vi "Producer:Consumer_UI.vi"() -> ()   [LabVIEW 2023]
panel:
  out "평가 데이터":string
  out "분석 데이터":bool
  out "측정 데이터":i32[](array[numeric])
  in  "종료":bool
  in  "평가":bool
  in  "분석":bool
  in  "측정":bool
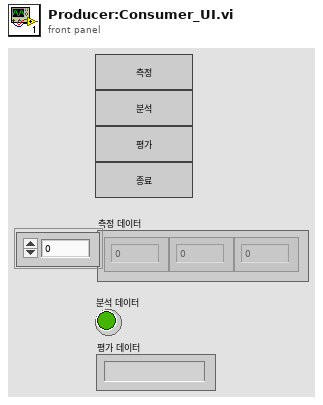
[diagram p1: front panel]
types:
  T1 = typedef "상태.ctl" = enum16{"측정", "분석", "평가", "종료"}
  T2 = enum8{"Enabled", "Disabled", "Disabled and Grayed Out"}
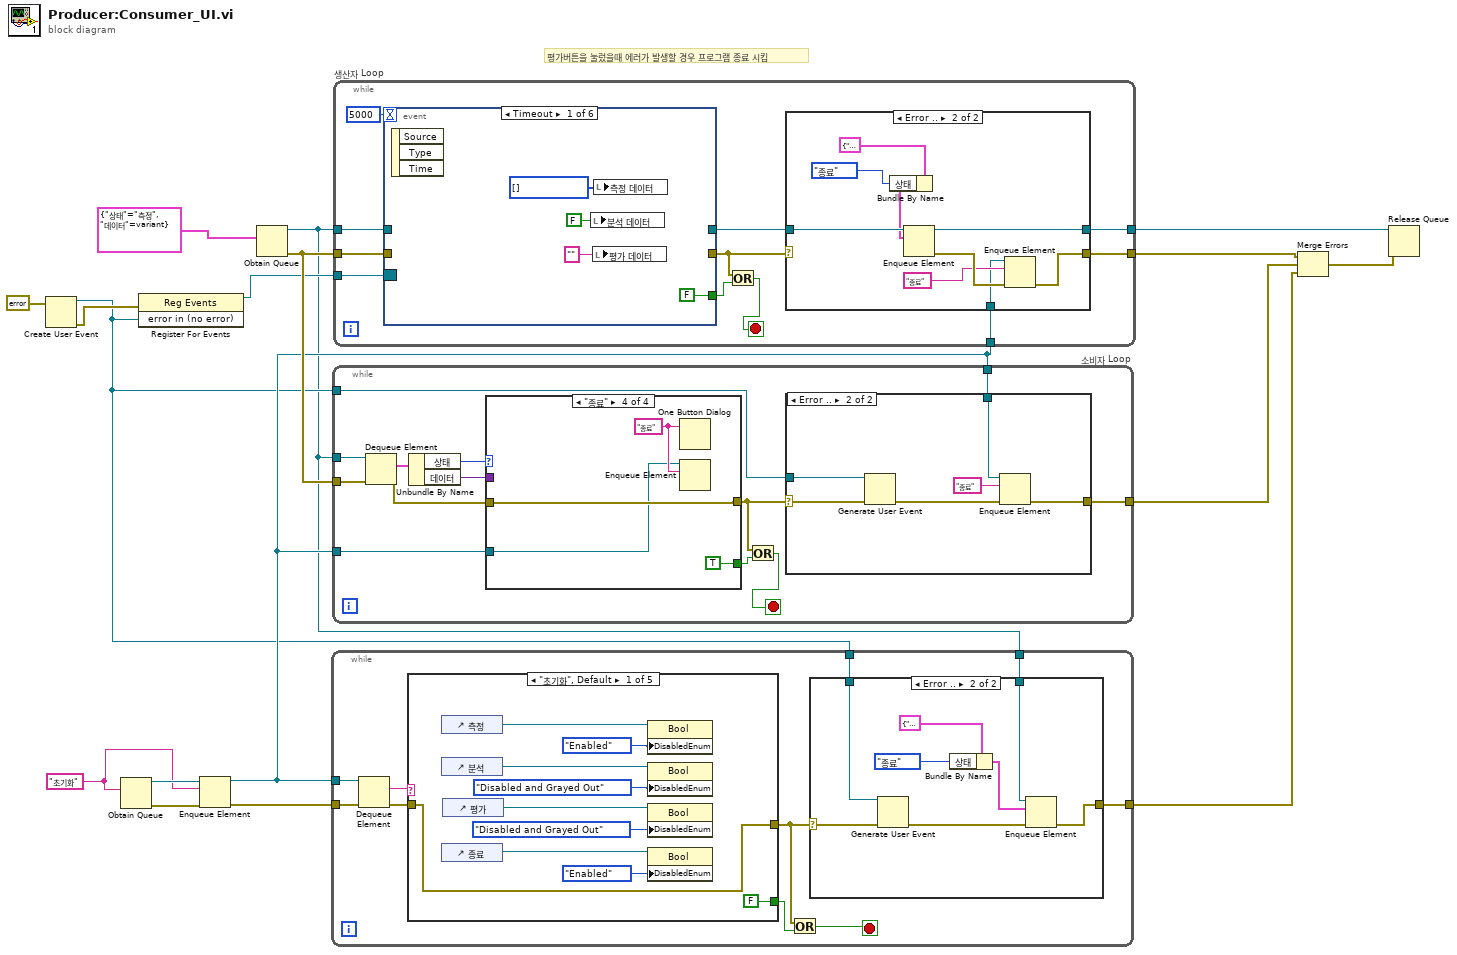
[diagram p0: block diagram]
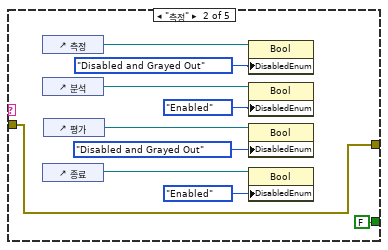
[diagram p3: hidden frame]
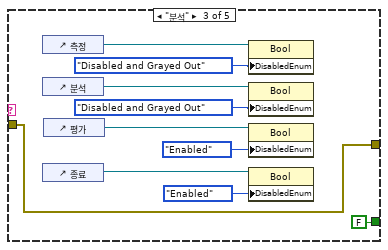
[diagram p4: hidden frame]
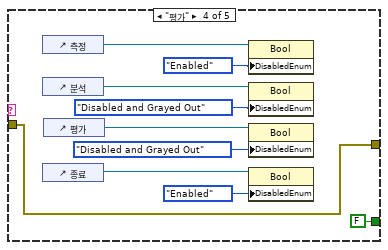
[diagram p5: hidden frame]
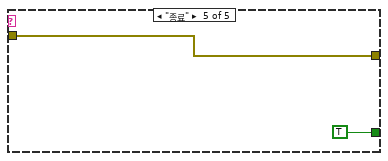
[diagram p6: hidden frame]
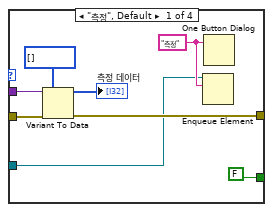
[diagram p8: hidden frame]
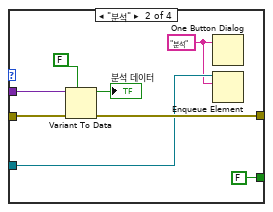
[diagram p9: hidden frame]
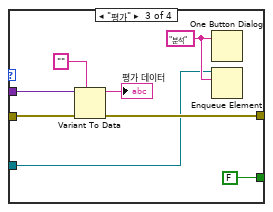
[diagram p10: hidden frame]
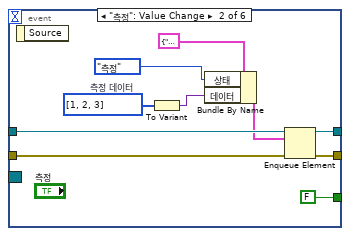
[diagram p12: hidden frame]
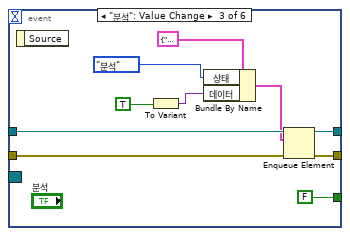
[diagram p13: hidden frame]
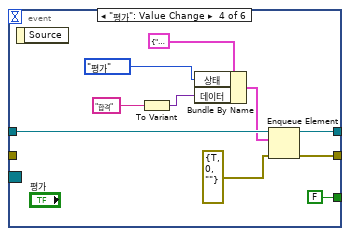
[diagram p14: hidden frame]
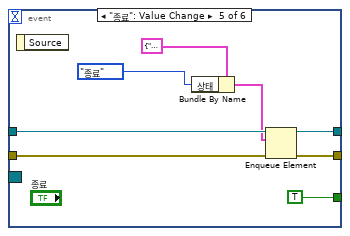
[diagram p15: hidden frame]
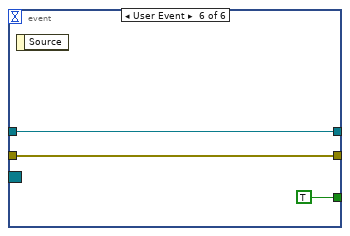
[diagram p16: hidden frame]
diagram:
  w1 = "초기화" ("name (unnamed)")
  # "평가버튼을 눌렀을때 에러가 발생할 경우 프로그램 종료 시킴"
  n1 = Create User Event(user event datatype=errorcluster {"status"=FALSE, "code"=0, "source"=""} ("error in (no error)")) -> (user event=w3:refnum<user-event>, error out=w10:errorcluster)  [unwired: 1 in]
  n2 = Obtain Queue(element data type=w1) -> (queue out=w8:refnum<queue>, error out=w7:errorcluster)  [unwired: 4 in, 1 out]
  n3 = register-events(error in=w10, w3) -> (reference out=w9:refnum<event-registration>)  [unwired: 1 in, 1 out]
  n4 = Enqueue Element(queue=w8, element=w1, error in (no error)=w7) -> (queue out=w4:refnum<queue>, error out=w6:errorcluster)  [unwired: 1 in, 1 out]
  n5 = Obtain Queue(element data type=cluster{"상태":T1, "데이터":variant} {"상태"=enum."측정", "데이터"=variant}) -> (queue out=w2:refnum<queue>, error out=w17:errorcluster)  [unwired: 4 in, 1 out]
  n6 = while {
    tunnel: w4 -> [w27]
    tunnel: w6 -> [w26]
    tunnel: [w19] -> w5
    tunnel: w3 -> [w20]
    tunnel: w2 -> [w18]
    stop <- w23 stop-if-true
    n7 = Dequeue Element(queue=w27, error in (no error)=w26) -> (element=w25:string, error out=w24:errorcluster)  [unwired: 1 in, 2 out]
    n8 = case shown="\"초기화\", Default" w25 {
      tunnel: [FALSE FALSE FALSE FALSE TRUE] -> w22
      tunnel: [w37 w47 w57 w67 w77] -> w21
      tunnel: w24 -> [w37 w47 w57 w67 w77]
      frame "초기화", Default {
        n9 = control-ref of="측정"() -> (w46:refnum<vi>)
        n10 = control-ref of="분석"() -> (w45:refnum<vi>)
        n11 = control-ref of="종료"() -> (w43:refnum<vi>)
        n12 = control-ref of="평가"() -> (w44:refnum<vi>)
        n13 = property class="Bool"(reference=w46, "DisabledEnum"=T2."Enabled" ("Disabled")) -> ()  [unwired: 1 in, 2 out]
        n14 = property class="Bool"(reference=w45, "DisabledEnum"=T2."Disabled and Grayed Out" ("Disabled")) -> ()  [unwired: 1 in, 2 out]
        n15 = property class="Bool"(reference=w44, "DisabledEnum"=T2."Disabled and Grayed Out" ("Disabled")) -> ()  [unwired: 1 in, 2 out]
        n16 = property class="Bool"(reference=w43, "DisabledEnum"=T2."Enabled" ("Disabled")) -> ()  [unwired: 1 in, 2 out]
      }
      frame "측정" {
        n17 = control-ref of="측정"() -> (w56:refnum<vi>)
        n18 = control-ref of="분석"() -> (w55:refnum<vi>)
        n19 = control-ref of="종료"() -> (w53:refnum<vi>)
        n20 = control-ref of="평가"() -> (w54:refnum<vi>)
        n21 = property class="Bool"(reference=w56, "DisabledEnum"=T2."Disabled and Grayed Out" ("Disabled")) -> ()  [unwired: 1 in, 2 out]
        n22 = property class="Bool"(reference=w55, "DisabledEnum"=T2."Enabled" ("Disabled")) -> ()  [unwired: 1 in, 2 out]
        n23 = property class="Bool"(reference=w54, "DisabledEnum"=T2."Disabled and Grayed Out" ("Disabled")) -> ()  [unwired: 1 in, 2 out]
        n24 = property class="Bool"(reference=w53, "DisabledEnum"=T2."Enabled" ("Disabled")) -> ()  [unwired: 1 in, 2 out]
      }
      frame "분석" {
        n25 = control-ref of="측정"() -> (w66:refnum<vi>)
        n26 = control-ref of="분석"() -> (w65:refnum<vi>)
        n27 = control-ref of="종료"() -> (w63:refnum<vi>)
        n28 = control-ref of="평가"() -> (w64:refnum<vi>)
        n29 = property class="Bool"(reference=w66, "DisabledEnum"=T2."Disabled and Grayed Out" ("Disabled")) -> ()  [unwired: 1 in, 2 out]
        n30 = property class="Bool"(reference=w65, "DisabledEnum"=T2."Disabled and Grayed Out" ("Disabled")) -> ()  [unwired: 1 in, 2 out]
        n31 = property class="Bool"(reference=w64, "DisabledEnum"=T2."Enabled" ("Disabled")) -> ()  [unwired: 1 in, 2 out]
        n32 = property class="Bool"(reference=w63, "DisabledEnum"=T2."Enabled" ("Disabled")) -> ()  [unwired: 1 in, 2 out]
      }
      frame "평가" {
        n33 = control-ref of="측정"() -> (w76:refnum<vi>)
        n34 = control-ref of="분석"() -> (w75:refnum<vi>)
        n35 = control-ref of="종료"() -> (w73:refnum<vi>)
        n36 = control-ref of="평가"() -> (w74:refnum<vi>)
        n37 = property class="Bool"(reference=w76, "DisabledEnum"=T2."Enabled" ("Disabled")) -> ()  [unwired: 1 in, 2 out]
        n38 = property class="Bool"(reference=w75, "DisabledEnum"=T2."Disabled and Grayed Out" ("Disabled")) -> ()  [unwired: 1 in, 2 out]
        n39 = property class="Bool"(reference=w74, "DisabledEnum"=T2."Disabled and Grayed Out" ("Disabled")) -> ()  [unwired: 1 in, 2 out]
        n40 = property class="Bool"(reference=w73, "DisabledEnum"=T2."Enabled" ("Disabled")) -> ()  [unwired: 1 in, 2 out]
      }
      frame "종료" {
      }
    }
    n41 = Or(x=w21, y=w22) -> (x .or. y?=w23:bool)
    n42 = case shown="Error .." w21 {
      selector: w21 -> [w28 w30]
      tunnel: w20 -> [_ w29]
      tunnel: [w28 w33] -> w19
      tunnel: w18 -> [_ w32]
      frame No Error {
      }
      frame Error {
        n43 = Generate User Event(user event=w29, error in=w30) -> (error out=w31:errorcluster)  [unwired: 2 in, 1 out]
        n44 = Bundle By Name(cluster=cluster{"상태":T1, "데이터":variant} {"상태"=enum."측정", "데이터"=variant}, "상태"=상태."종료") -> (w34:cluster{"상태":T1, "데이터":variant})
        n45 = Enqueue Element(queue=w32, element=w34, error in (no error)=w31) -> (error out=w33:errorcluster)  [unwired: 1 in, 2 out]
      }
    }
  }
  n46 = while "소비자 Loop" {
    tunnel: w2 -> [w91]
    tunnel: w17 -> [w90]
    tunnel: [w81] -> w14
    tunnel: w3 -> [w82]
    tunnel: w4 -> [w80]
    tunnel: w4 -> [w79]
    stop <- w84 stop-if-true
    n47 = Dequeue Element(queue=w91, error in (no error)=w90) -> (element=w89:cluster{"상태":T1, "데이터":variant}, error out=w86:errorcluster)  [unwired: 1 in, 2 out]
    n48 = Unbundle By Name(w89) -> ("상태"=w88:T1, "데이터"=w87:variant)
    n49 = case shown="\"종료\"" w88 {
      tunnel: w87 -> [w106 w114 w122 _]
      tunnel: [FALSE FALSE FALSE TRUE] -> w85
      tunnel: w86 -> [w102 w110 w118 w125]
      tunnel: [w101 w109 w117 w125] -> w83
      tunnel: w80 -> [w99 w108 w115 w123]
      frame "측정", Default {
        w100 = "측정" ("message")
        n50 = Variant To Data(error in=w102, type=i32[] [] ("측정 데이터"), Variant=w106) -> (data=→"측정 데이터":i32[], error out=w101:errorcluster)
        n51 = Enqueue Element(queue=w99, element=w100) -> ()  [unwired: 2 in, 3 out]
        n52 = One Button Dialog(message=w100) -> ()  [unwired: 1 in, 1 out]
      }
      frame "분석" {
        w107 = "분석" ("message")
        n53 = Variant To Data(error in=w110, type=FALSE ("분석 데이터"), Variant=w114) -> (data=→"분석 데이터":bool, error out=w109:errorcluster)
        n54 = One Button Dialog(message=w107) -> ()  [unwired: 1 in, 1 out]
        n55 = Enqueue Element(queue=w108, element=w107) -> ()  [unwired: 2 in, 3 out]
      }
      frame "평가" {
        w116 = "분석" ("message")
        n56 = Variant To Data(error in=w118, type="" ("평가 데이터"), Variant=w122) -> (data=→"평가 데이터":string, error out=w117:errorcluster)
        n57 = One Button Dialog(message=w116) -> ()  [unwired: 1 in, 1 out]
        n58 = Enqueue Element(queue=w115, element=w116) -> ()  [unwired: 2 in, 3 out]
      }
      frame "종료" {
        w124 = "종료" ("message")
        n59 = One Button Dialog(message=w124) -> ()  [unwired: 1 in, 1 out]
        n60 = Enqueue Element(queue=w123, element=w124) -> ()  [unwired: 2 in, 3 out]
      }
    }
    n61 = Or(x=w83, y=w85) -> (x .or. y?=w84:bool)
    n62 = case shown="Error .." w83 {
      selector: w83 -> [w92 w98]
      tunnel: w82 -> [_ w97]
      tunnel: [w92 w94] -> w81
      tunnel: w79 -> [_ w96]
      frame No Error {
      }
      frame Error {
        n63 = Generate User Event(user event=w97, event data cluster=w98) -> (error out=w95:errorcluster)  [unwired: 2 in, 1 out]
        n64 = Enqueue Element(queue=w96, element="종료", error in (no error)=w95) -> (error out=w94:errorcluster)  [unwired: 1 in, 2 out]
      }
    }
  }
  n65 = while "생산자 Loop" {
    tunnel: w17 -> [w137]
    tunnel: w2 -> [w136]
    tunnel: [w130] -> w13
    tunnel: [w129] -> w12
    tunnel: w9 -> [w128]
    tunnel: w4 -> [w127]
    stop <- w133 stop-if-true
    n66 = event shown="[0] Timeout" {
      selector: w128 -> [_ _ _ _ _ _]
      dyn-events: _ -> [_ _ _ _ _ _]
      timeout: 5000 -> [_ _ _ _ _ _]
      tunnel: w137 -> [_ w162 w166 _ w186 w191]
      tunnel: [_ w161 w167 w180 w185 w191] -> w132
      tunnel: w136 -> [_ w160 w169 w182 w188 w192]
      tunnel: [_ w159 w168 w181 w187 _] -> w131
      tunnel: [FALSE FALSE FALSE FALSE TRUE TRUE] -> w134
      tunnel: [_ _ _ _ _ w192] -> _
      event Timeout {
        n67 = event-data() -> ()  [unwired: 1 in, 3 out]
        n68 = local write "분석 데이터"(FALSE ("분석 데이터")) -> ()
        n69 = local write "평가 데이터"("" ("평가 데이터")) -> ()
        n70 = local write "측정 데이터"(i32[] [] ("측정 데이터")) -> ()
      }
      event "측정": Value Change {
        w155 = i32[] [1, 2, 3]  # 측정 데이터
        n71 = event-data() -> ()  [unwired: 1 in, 1 out]
        n72 = To Variant(anything=w155) -> (Variant=w156:variant)
        n73 = Bundle By Name(cluster=cluster{"상태":T1, "데이터":variant} {"상태"=enum."측정", "데이터"=variant}, "상태"=상태."측정", "데이터"=w156) -> (w154:cluster{"상태":T1, "데이터":variant})
        n74 = Enqueue Element(queue=w160, element=w154, error in (no error)=w162) -> (queue out=w159:refnum<queue>, error out=w161:errorcluster)  [unwired: 1 in, 1 out]
      }
      event "분석": Value Change {
        n75 = event-data() -> ()  [unwired: 1 in, 1 out]
        n76 = To Variant(anything=TRUE ("분석 데이터")) -> (Variant=w170:variant)
        n77 = Bundle By Name(cluster=cluster{"상태":T1, "데이터":variant} {"상태"=enum."측정", "데이터"=variant}, "상태"=상태."분석", "데이터"=w170) -> (w164:cluster{"상태":T1, "데이터":variant})
        n78 = Enqueue Element(queue=w169, element=w164, error in (no error)=w166) -> (queue out=w168:refnum<queue>, error out=w167:errorcluster)  [unwired: 1 in, 1 out]
      }
      event "평가": Value Change {
        n79 = event-data() -> ()  [unwired: 1 in, 1 out]
        n80 = To Variant(anything="합격" ("평가 데이터")) -> (Variant=w177:variant)
        n81 = Bundle By Name(cluster=cluster{"상태":T1, "데이터":variant} {"상태"=enum."측정", "데이터"=variant}, "상태"=상태."평가", "데이터"=w177) -> (w176:cluster{"상태":T1, "데이터":variant})
        n82 = Enqueue Element(queue=w182, element=w176, error in (no error)=errorcluster {"status"=TRUE, "code"=0, "source"=""}) -> (queue out=w181:refnum<queue>, error out=w180:errorcluster)  [unwired: 1 in, 1 out]
      }
      event "종료": Value Change {
        n83 = event-data() -> ()  [unwired: 1 in, 1 out]
        n84 = Bundle By Name(cluster=cluster{"상태":T1, "데이터":variant} {"상태"=enum."측정", "데이터"=variant}, "상태"=상태."종료") -> (w184:cluster{"상태":T1, "데이터":variant})
        n85 = Enqueue Element(queue=w188, element=w184, error in (no error)=w186) -> (queue out=w187:refnum<queue>, error out=w185:errorcluster)  [unwired: 1 in, 1 out]
      }
      event User Event {
        n86 = event-data() -> ()  [unwired: 1 in, 1 out]
      }
    }
    n87 = Or(x=w132, y=w134) -> (x .or. y?=w133:bool)
    n88 = case shown="Error .." w132 {
      selector: w132 -> [w138 _]
      tunnel: w131 -> [w139 w146]
      tunnel: [w139 w145] -> w130
      tunnel: [w138 w142] -> w129
      tunnel: w127 -> [_ w140]
      frame No Error {
      }
      frame Error {
        n89 = Bundle By Name(cluster=cluster{"상태":T1, "데이터":variant} {"상태"=enum."측정", "데이터"=variant}, "상태"=상태."종료") -> (w144:cluster{"상태":T1, "데이터":variant})
        n90 = Enqueue Element(queue=w146, element=w144) -> (queue out=w145:refnum<queue>, error out=w143:errorcluster)  [unwired: 2 in, 1 out]
        n91 = Enqueue Element(queue=w140, element="종료", error in (no error)=w143) -> (error out=w142:errorcluster)  [unwired: 1 in, 2 out]
      }
    }
  }
  n92 = Merge Errors(w12, w14, w5) -> (w15:errorcluster)
  n93 = Release Queue(queue=w13, error in (no error)=w15) -> ()  [unwired: 1 in, 3 out]
